vi "Read In.vi"(1 "File path":path=path "C:/Users/Marvin/Documents/SPLAT/nieuwe_data.txt") -> (0 "DataOut [tagID, anchorID, distance, time]":string[][](array[string]))   [LabVIEW 2014, in "Position.lvclass"]
uses:
  Position.lvclass
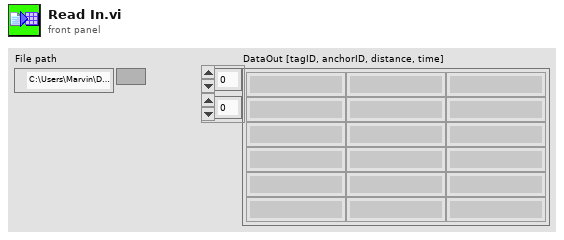
[diagram p1: front panel]
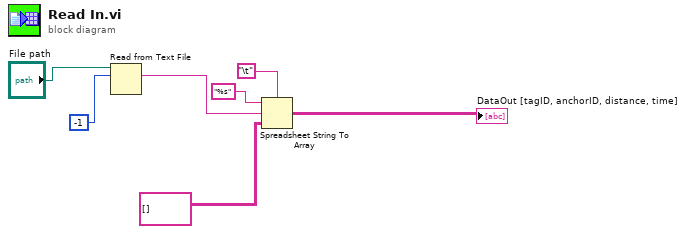
[diagram p0: block diagram]
diagram:
  n1 = Read from Text File(file (use dialog)="File path", count=-1) -> (text=w6:string)  [unwired: 2 in, 3 out]
  n2 = Spreadsheet String To Array(delimiter (Tab)="\t", format string="%s", spreadsheet string=w6, array type (2D Dbl)=string[][] []) -> (array=→"DataOut [tagID, anchorID, distance, time]":string[][])
